vi "SpiralPoints-FixedAngle.vi"(0 "m: Number of spirals/turn":u16=3 min=1, 1 "a: Pitch (minimal distace)":dbl=505.0, 2 "r0: Start Radius":dbl=47100.0, 3 "width (<<r0)":dbl=14400.0, 4 "Track density (here only 1)":dbl=1.0 min=1e-06) -> (5 "Coordinates":cdb[](array[numeric]), 6 "imax: number of points per spiral":dbl=541.0)   [LabVIEW 2011]
panel:
  out "nmax":dbl
  out "k1":dbl
  out "APitch":dbl
  out "radialPitchStart":dbl
  out "N per turn":dbl
  out "XY Graph":cluster{dbl, dbl}[](graph)
  # "Pattern is Andromeda-type"
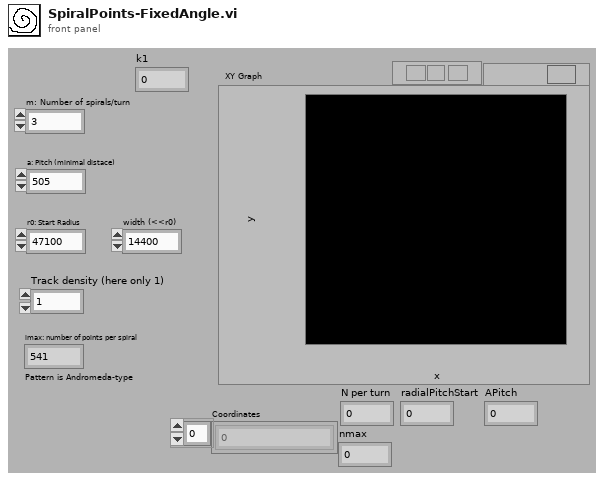
[diagram p1: front panel]
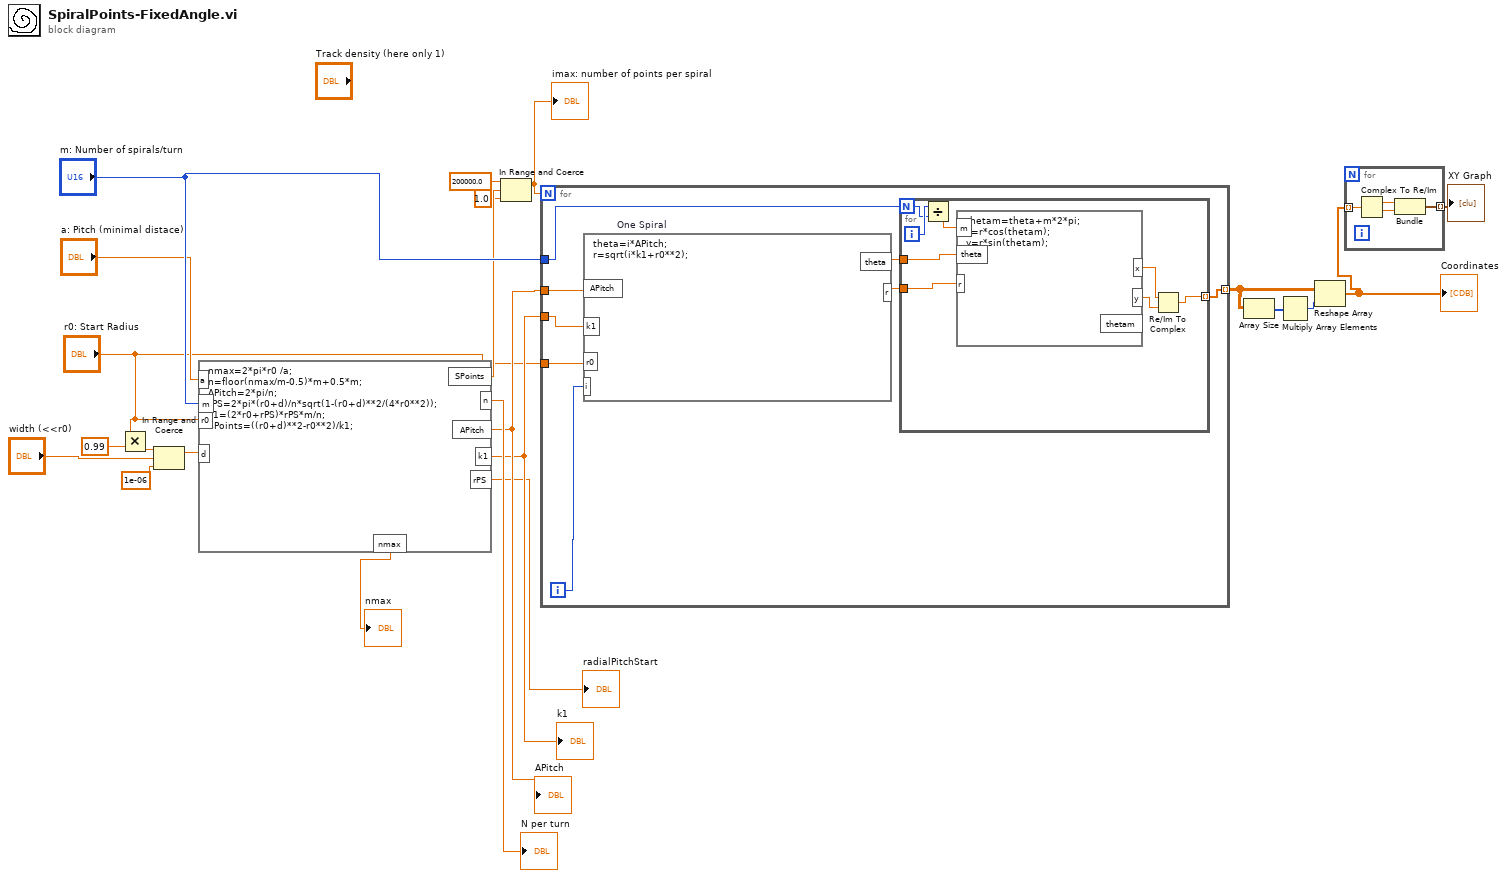
[diagram p0: block diagram]
diagram:
  n1 = Multiply(x="r0: Start Radius", y=0.99) -> (x*y=w2:dbl)
  n2 = In Range and Coerce(upper limit=w2, x="width (<<r0)", lower limit=1e-06) -> (coerced(x)=w6:dbl)  [unwired: 1 out]
  n3 = formula code="nmax=2*pi*r0 /a;\nn=floor(nmax/m-0.5)*m+0.5*m;\nAPitch=2*pi/n;\nrPS=2*pi*(r0+d)/n*sqrt(1-(r0+d)**2/(4*r0**2));\nk1=(2*r0+rPS)*rPS*m/n;\nSPoints=((r0+d)**2-r0**2)/k1;"("r0"="r0: Start Radius", "d"=w6, "a"="a: Pitch (minimal distace)", "m"="m: Number of spirals/turn") -> ("n"=→"N per turn":dbl, "nmax"=→"nmax":dbl, "APitch"=w14:dbl, "k1"=w13:dbl, "rPS"=→"radialPitchStart":dbl, "SPoints"=w10:dbl)
  "APitch" <- w14
  "k1" <- w13
  n4 = In Range and Coerce(upper limit=200000.0, x=w10, lower limit=1.0) -> (coerced(x)=w9:dbl)  [unwired: 1 out]
  "imax: number of points per spiral" <- w9
  n5 = for {
    N: w9 -> [_]
    tunnel: "m: Number of spirals/turn" -> [w26]
    tunnel: w14 -> [w30]
    tunnel: "r0: Start Radius" -> [w29]
    tunnel: [w25] -> w22 mode=indexing
    tunnel: w13 -> [w24]
    i -> [w23]
    n6 = formula code="theta=i*APitch;\nr=sqrt(i*k1+r0**2);" "One Spiral"("APitch"=w30, "i"=w23, "r0"=w29, "k1"=w24) -> ("theta"=w28:dbl, "r"=w27:dbl)
    n7 = for {
      N: w26 -> [w36]
      tunnel: [w31] -> w25 mode=indexing
      tunnel: w28 -> [w38]
      tunnel: w27 -> [w34]
      i -> [w37]
      n8 = Divide(x=w37, y=w36) -> (x/y=w35:dbl)
      n9 = formula code="thetam=theta+m*2*pi;\nx=r*cos(thetam);\ny=r*sin(thetam);"("theta"=w38, "r"=w34, "m"=w35) -> ("x"=w33:dbl, "y"=w32:dbl)  [unwired: 1 out]
      n10 = Re/Im To Complex(1:w32, 2:w33) -> (0:w31:cdb)
    }
  }
  n11 = Array Size(array=w22) -> (size(s)=w20:i32[])
  n12 = Multiply Array Elements(1:w20) -> (0:w21:i32)
  n13 = Reshape Array(w22, w21) -> (w16:cdb[])
  "Coordinates" <- w16
  n14 = for {
    tunnel: w16 -> [w42] mode=indexing
    tunnel: [w39] -> w15 mode=indexing
    n15 = Complex To Re/Im(x + iy=w42) -> (x=w41:dbl, y=w40:dbl)
    n16 = Bundle(w41, w40) -> (w39:cluster{dbl, dbl})  [unwired: 1 out]
  }
  "XY Graph" <- w15
